vi "LS 340 check temp stability.vi"(7 "Set point proximity":dbl=0.05 format="%.3f", 8 "error in (no error)":errorcluster, 9 "seconds to wait":i32=30, 10 "Stability":dbl=0.05 format="%.3f", 11 "VISA Resource Name":refnum<visa-resource-name>) -> (0 "error out":errorcluster, 3 "VISA Resource Name Out":refnum<visa-resource-name>)   [LabVIEW 2015]
panel:
  out "Temperature":dbl=26.719 format="%.4f"
  out "Waveform Chart":dbl(graph)=26.719
  out "Set Point":dbl=40.0 format="%.4f"
  in  "Sample time Secs":dbl=1.0
  # "Checking for temperature stability"
  # "Temperature must be within +/-"
  # "of set point"
  # "and stable within +/-"
  # "over"
  # "Seconds"
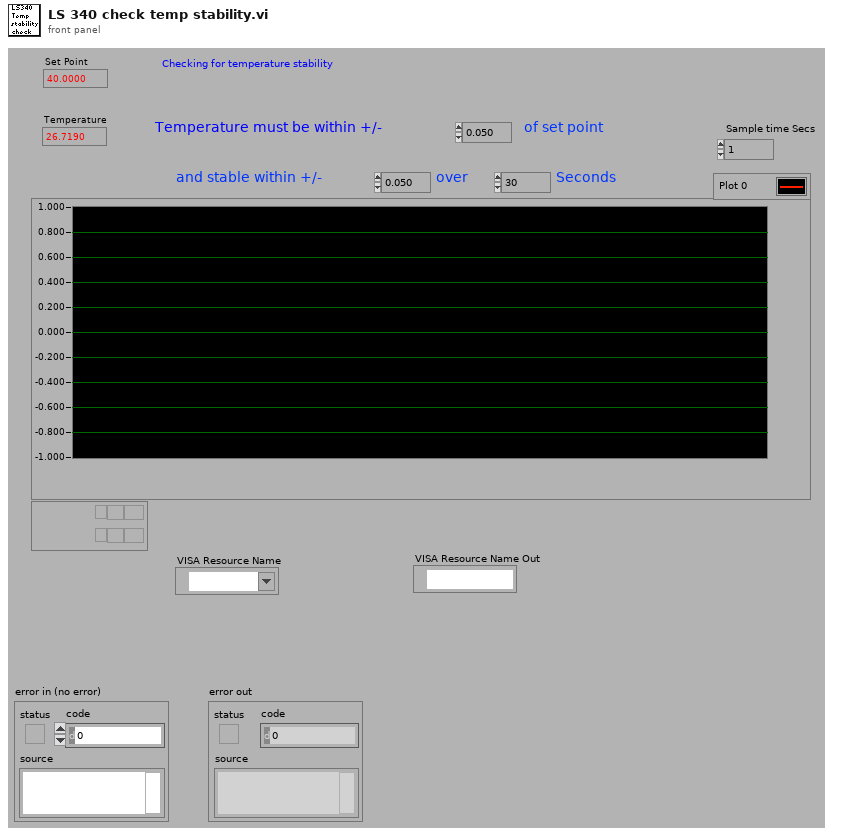
[diagram p1: front panel]
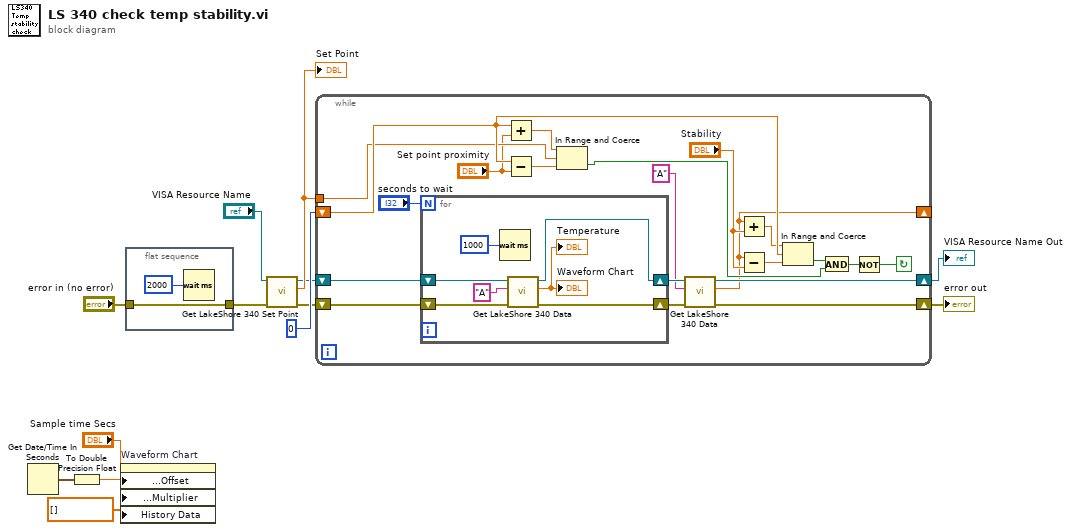
[diagram p0: block diagram]
diagram:
  n1 = Get Date/Time In Seconds() -> (seconds since 1Jan1904=w5:timestamp)
  n2 = To Double Precision Float(number=w5) -> (double precision float=w8:dbl)
  n3 = property on="Waveform Chart" class="WFChart (strict)"("X Scale.Offset and Multiplier:Offset"=w8, "X Scale.Offset and Multiplier:Multiplier"="Sample time Secs", "History Data"=dbl[] [] ("Write Attribute")) -> ()  [unwired: 2 in, 2 out]
  n4 = flat-sequence {
    tunnel: "error in (no error)" -> [w14]
    tunnel: [w14] -> w3
    frame #0 {
      n5 = Wait (ms)(milliseconds to wait=u32 2000) -> ()  [unwired: 1 out]
    }
  }
  n6 = call "Get LakeShore 340 Set Point.vi"("error in (no error)"=w3, "VISA Resource Name"="VISA Resource Name") -> ("error out"=w9:errorcluster, "Set point"=w11:dbl, "VISA Resource Name Out"=w10:refnum<visa-resource-name>)  [unwired: 7 in]
  "Set Point" <- w11
  n7 = while {
    tunnel: w11 -> [w34]
    shift-left: 0 -> [w35]
    shift-right: [w18] -> _
    shift-right: [w32] -> w1
    shift-left: w10 -> [w33]
    shift-right: [w17] -> w2
    shift-left: w9 -> [w16]
    stop <- w36 continue-if-true
    n8 = for {
      N: "seconds to wait" -> [_]
      shift-right: [w40] -> w21
      shift-left: w33 -> [w42]
      shift-right: [w38] -> w20
      shift-left: w16 -> [w37]
      n9 = Wait (ms)(milliseconds to wait=u32 1000) -> ()  [unwired: 1 out]
      n10 = call "Get LakeShore 340 Data.vi"("error in (no error)"=w37, "Input (A or B)"="A", "VISA Resource Name"=w42) -> ("error out"=w38:errorcluster, "Temperature"=→"Temperature" →"Waveform Chart":dbl, "VISA Resource Name Out"=w40:refnum<visa-resource-name>)  [unwired: 6 out]
    }
    n11 = Add(x=w35, y="Set point proximity") -> (x+y=w28:dbl)
    n12 = Subtract(x=w35, y="Set point proximity") -> (x-y=w27:dbl)
    n13 = In Range and Coerce(upper limit=w28, x=w34, lower limit=w27) -> (In Range?=w26:bool)  [unwired: 1 out]
    n14 = call "Get LakeShore 340 Data.vi"("error in (no error)"=w20, "Input (A or B)"="A", "VISA Resource Name"=w21) -> ("error out"=w17:errorcluster, "Temperature"=w18:dbl, "VISA Resource Name Out"=w32:refnum<visa-resource-name>)  [unwired: 6 out]
    n15 = Add(x=w18, y="Stability") -> (x+y=w31:dbl)
    n16 = Subtract(x=w18, y="Stability") -> (x-y=w30:dbl)
    n17 = In Range and Coerce(upper limit=w31, x=w35, lower limit=w30) -> (In Range?=w24:bool)  [unwired: 1 out]
    n18 = And(x=w24, y=w26) -> (x .and. y?=w23:bool)
    n19 = Not(x=w23) -> (.not. x?=w36:bool)
  }
  "error out" <- w2
  "VISA Resource Name Out" <- w1
